vi "Video Stuff v04.vi"() -> ()   [LabVIEW 2009]
doc: "This example illustrates the use of a calibration grid to calibrate and correct an image for nonlinear distortion and accurate shape measurements.\n\nThis example loads the image of a calibration grid used to calibrate the system, learns the grid, then loads an image of parts acquired using the same setup. The example then corrects the image in two ways. The first method corrects the entire image and then measures the area of the coins. The second method corrects only the area of the coins and displays the difference in processing time."
uses:
  <vilib>/userDefined/High Color/IMAQdx.ctl
  <vilib>/vision/NI_Vision_Development_Module.lvlib
  <vilib>/vision/driver/NI_Vision_Acquisition_Software.lvlib
panel:
  out "appended array":dbl[](array[numeric])
  out "x-y":dbl[][](array[numeric])
  out "Array":i32[][](array[numeric])
  out "Small":T1(plugin-control)
  in  "Resolution":i32=36
  in  "Camera Name":T2="cam0"
  in  "Video Modes":i32(listbox)
  in  "stop":bool
  out "Live Video":T1(plugin-control)
  out "Buffer Number":u32
  in  "Red Range":cluster{"Lower value":i32, "Upper value":i32}={"Lower value"=240, "Upper value"=255}
  in  "Green Range":cluster{"Lower value":i32, "Upper value":i32}={"Lower value"=250, "Upper value"=255}
  in  "Blue Range":cluster{"Lower value":i32, "Upper value":i32}={"Lower value"=250, "Upper value"=255}
  in  "Color Mode":u16(ring) items=["RGB", "HSL", "HSV", "HSI"]
  out "Super Filter":T1(plugin-control)
  in  "Calibration File Path":path=path "C:/Documents and Settings/ekolker/My Documents/OGRE/to be synched/calibrationGrid.PNG"
  out "Top Image":T1(plugin-control) caption="Calibration Template"
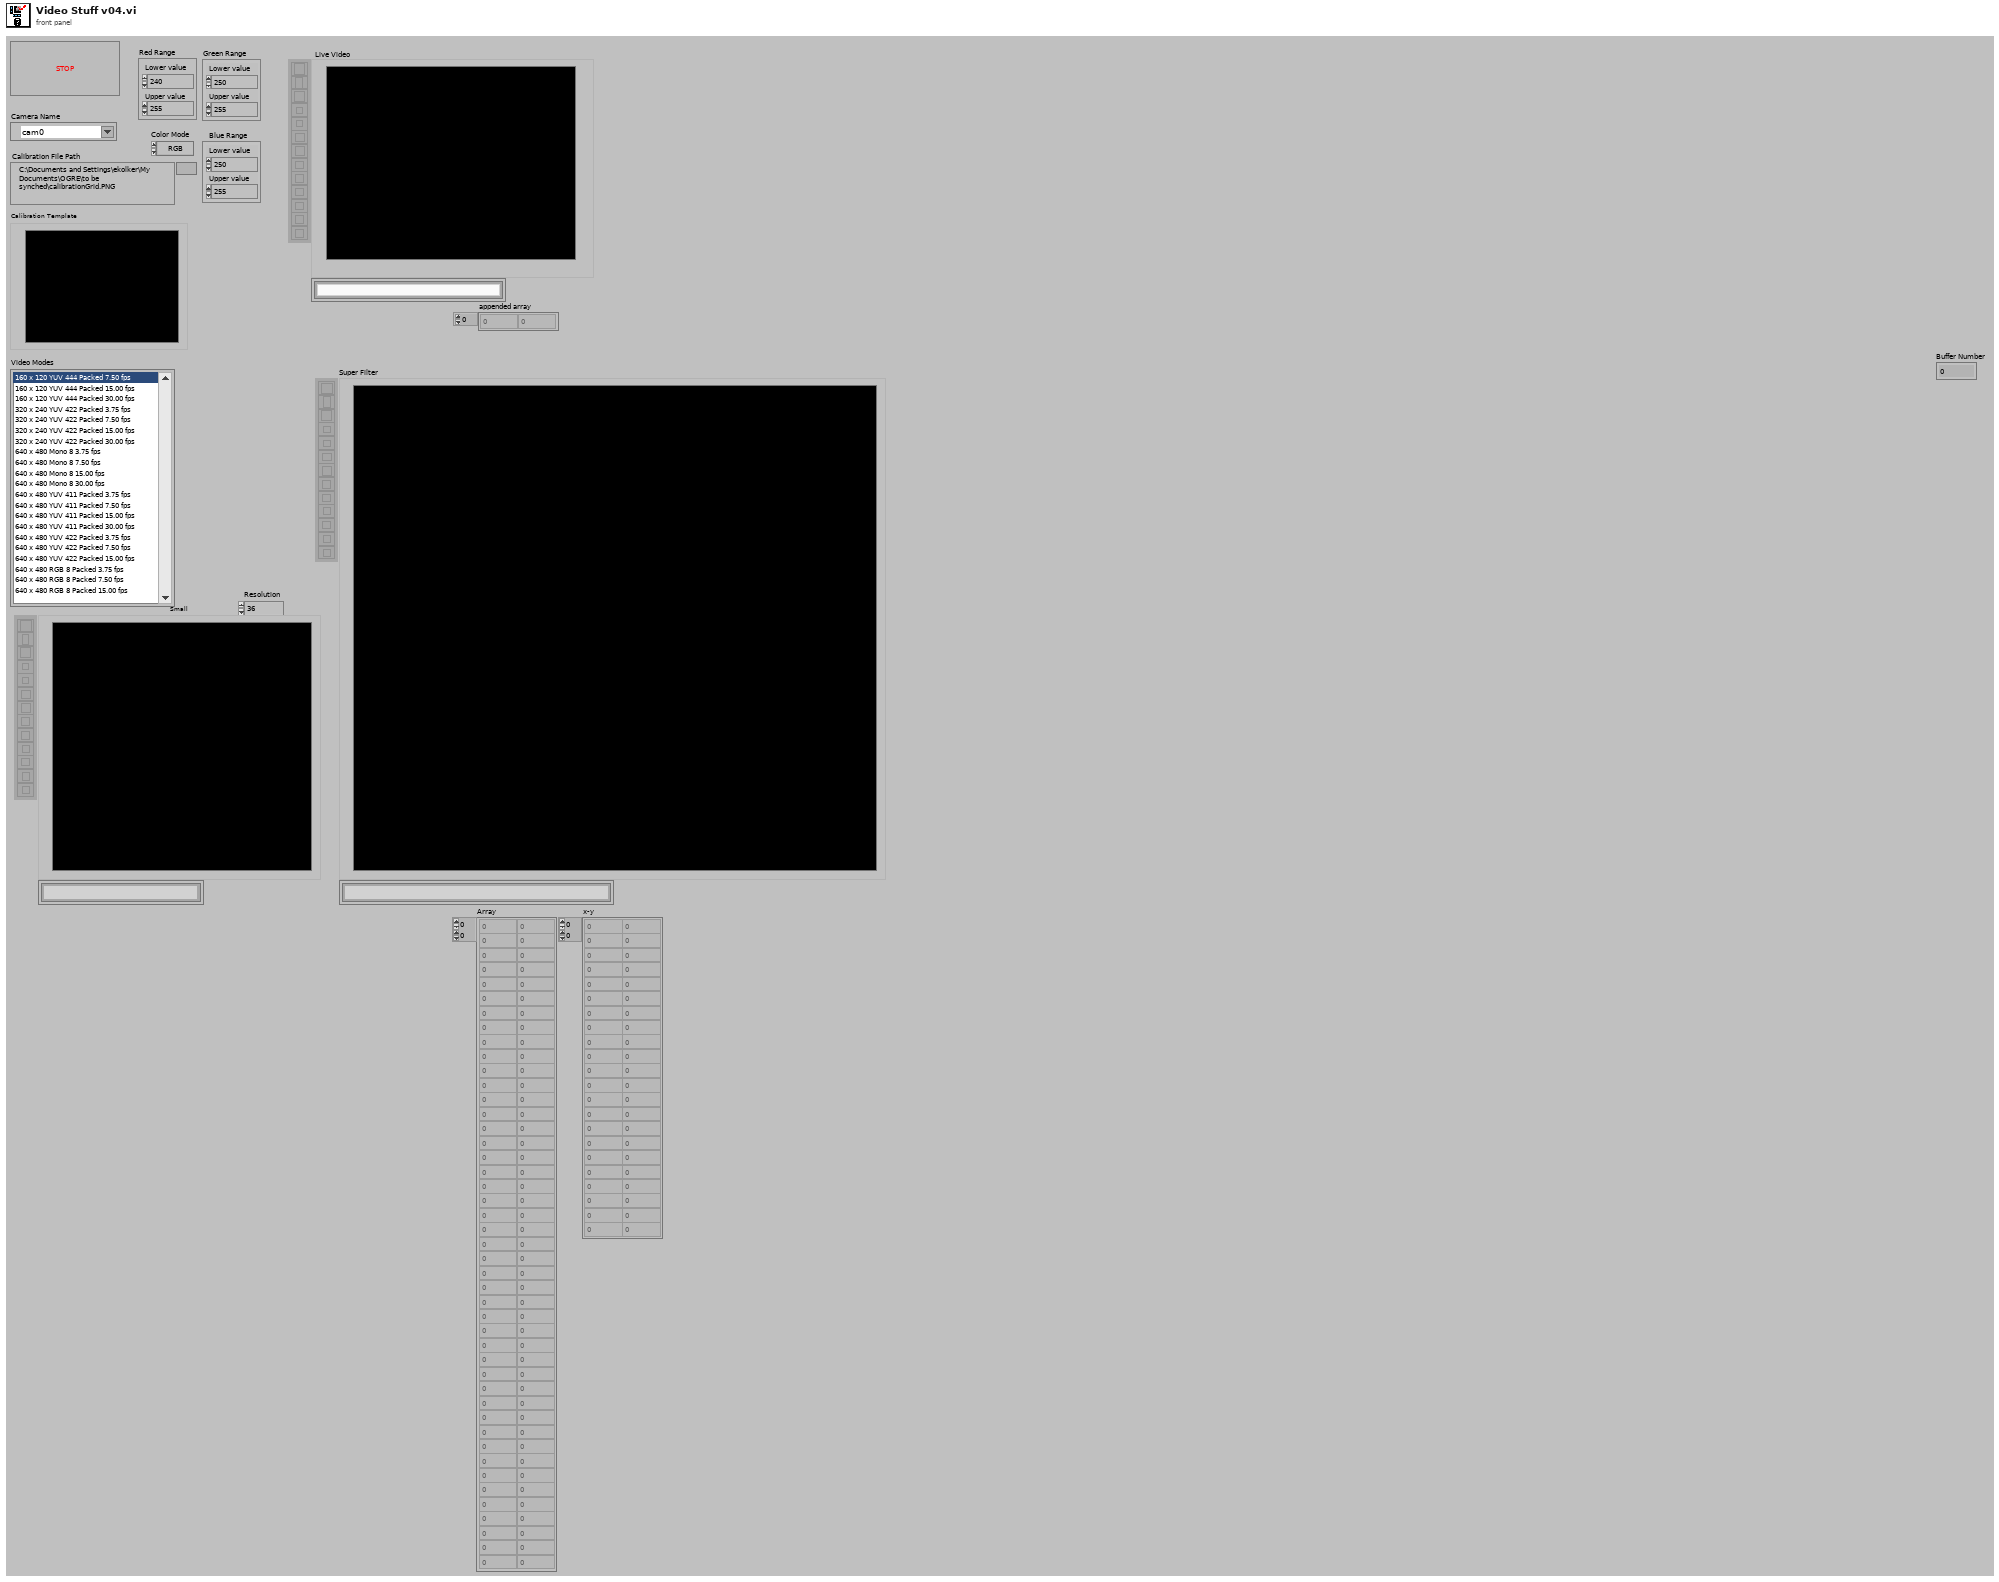
[diagram p1: front panel]
types:
  T1 = typedef "IMAQ Image.ctl" = refnum<image>
  T2 = typedef "IMAQdx.ctl" = refnum<k21>
  T3 = typedef "Image Type" = u32
  T4 = cluster{"X Step":sgl, "Y Step":sgl, "Unit":u32, "Threshold Range":cluster{"Lower value":sgl, "Upper value":sgl}}
  T5 = cluster{"Distortion":u32, "Corrected Image Scaling":u32, "Corrected Image Learn ROI":u32, "Learn Error Map?":bool, "Learn Correction Table?":bool}
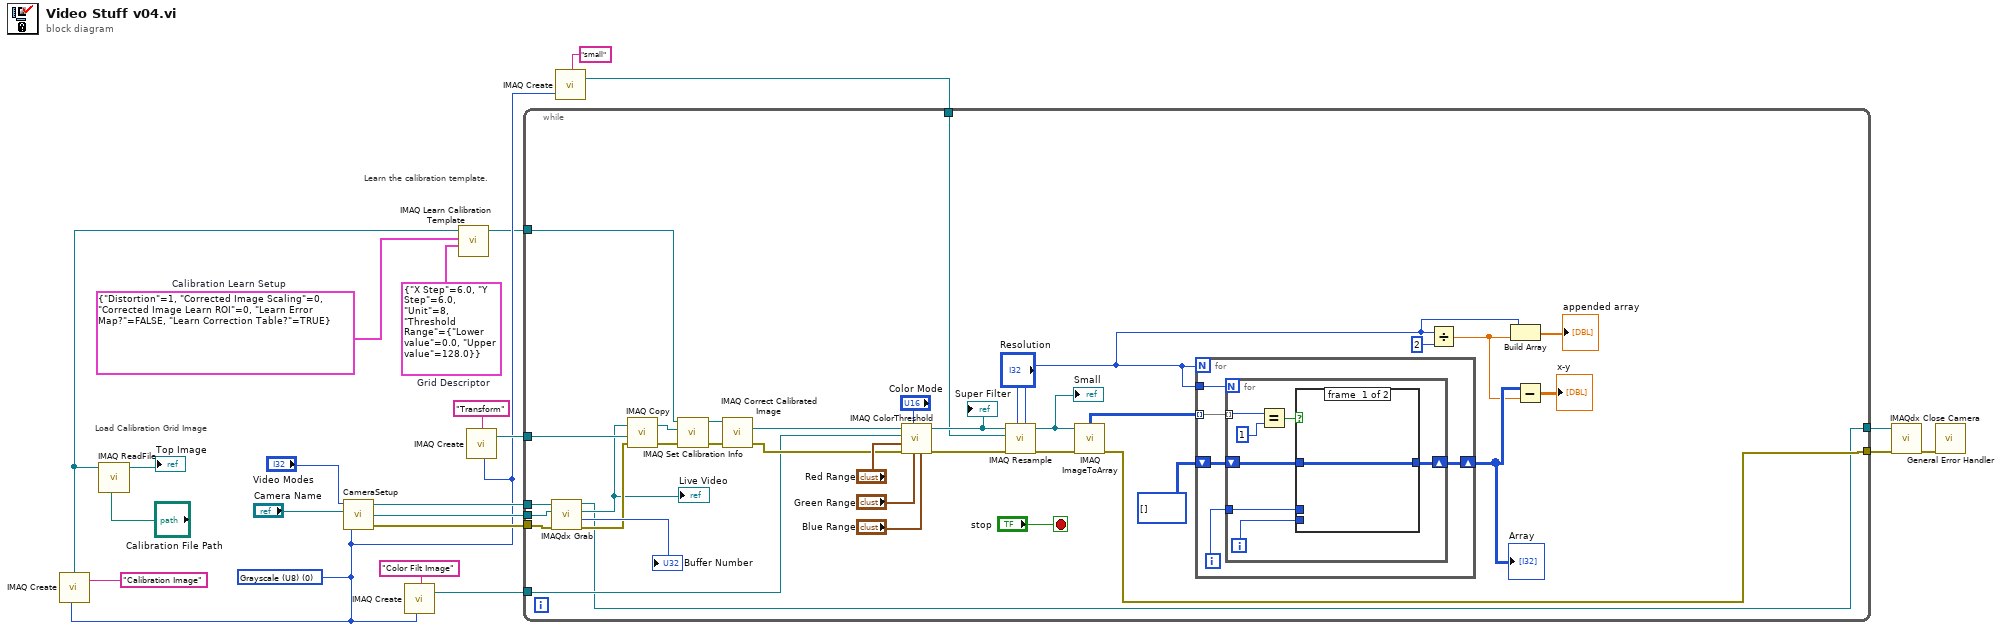
[diagram p0: block diagram]
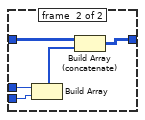
[diagram p2: hidden frame]
diagram:
  w3 = T3 0 items=["Grayscale (U8)", "Grayscale (I16)", "Grayscale (SGL)", "Complex (CSG)", "RGB (U32)", "HSL (U32)", "RGB (U64)", "Grayscale (U16)"] ("Image Type")
  w17 = T4 {"X Step"=6.0, "Y Step"=6.0, "Unit"=8, "Threshold Range"={"Lower value"=0.0, "Upper value"=128.0}}  # Grid Descriptor
  w18 = T5 {"Distortion"=1, "Corrected Image Scaling"=0, "Corrected Image Learn ROI"=0, "Learn Error Map?"=FALSE, "Learn Correction Table?"=TRUE}  # Calibration Learn Setup
  # "Load Calibration Grid Image"
  # "Learn the calibration template."
  n1 = call "IMAQ Create"("Image Name"="Calibration Image", "Image Type"=w3) -> ("New Image"=w2:T1)  [unwired: 2 in, 2 out]
  n2 = call "IMAQ ReadFile"("File Path"="Calibration File Path", "Image"=w2) -> ("Image Out"=→"Top Image":T1)  [unwired: 3 in, 6 out]
  n3 = call "CameraSetup.vi"("Image Type"=w3, "Camera Name"="Camera Name", "Video Modes"="Video Modes") -> ("error out"=w11:errorcluster, "New Image"=w6:T1, "Session Out"=w7:T2)  [unwired: 1 in]
  n4 = call "IMAQ Create"("Image Name"="Color Filt Image", "Image Type"=w3) -> ("New Image"=w20:T1)  [unwired: 2 in, 2 out]
  n5 = call "IMAQ Learn Calibration Template"("Grid Descriptor"=w17, "Calibration Learn Setup"=w18, "Image"=w2) -> ("Calibrated Image"=w1:T1)  [unwired: 4 in, 4 out]
  n6 = call "IMAQ Create"("Image Name"="Transform", "Image Type"=w3) -> ("New Image"=w19:T1)  [unwired: 2 in, 2 out]
  n7 = call "IMAQ Create"("Image Name"="small", "Image Type"=w3) -> ("New Image"=w9:T1)  [unwired: 2 in, 2 out]
  n8 = while {
    tunnel: w20 -> [w43]
    tunnel: [w30] -> w21
    tunnel: w19 -> [w49]
    tunnel: w11 -> [w44]
    tunnel: w9 -> [w31]
    tunnel: [w32] -> w8
    tunnel: w7 -> [w39]
    tunnel: w6 -> [w38]
    tunnel: w1 -> [w23]
    stop <- "stop" stop-if-true
    n9 = call <vilib>:"IMAQdx Grab.vi"("error in"=w44, "Image In"=w38, "Session In"=w39) -> ("error out"=w45:errorcluster, "Buffer Number Out"=→"Buffer Number":u32, "Image Out"=w42:T1, "Session Out"=w30:T2)  [unwired: 1 in, 4 out]
    "Live Video" <- w42
    n10 = call "IMAQ Copy"("error in (no error)"=w45, "Image Dst"=w49, "Image Src"=w42) -> ("error out"=w46:errorcluster, "Image Dst Out"=w51:T1)  [unwired: 3 in]
    n11 = call "IMAQ Set Calibration Info"("error in (no error)"=w46, "Image Dst"=w51, "Image Src"=w23) -> ("error out"=w47:errorcluster, "Calibrated Image"=w50:T1)  [unwired: 1 in, 6 out]
    n12 = call "IMAQ Correct Calibrated Image"("error in (no error)"=w47, "Image Src"=w50) -> ("error out"=w48:errorcluster, "Corrected Image"=w33:T1)  [unwired: 5 in, 3 out]
    n13 = call "IMAQ ColorThreshold"("Blue or Luma or Val or Inten Range"="Blue Range", "Green or Sat Range"="Green Range", "Color Mode"="Color Mode", "error in (no error)"=w48, "Red or Hue Range"="Red Range", "Image Dst"=w43, "Image Src"=w33) -> ("error out"=w41:errorcluster, "Image Dst Out"=w40:T1)  [unwired: 3 in]
    "Super Filter" <- w40
    n14 = call "IMAQ Resample"("X Resolution"="Resolution", "Y Resolution"="Resolution", "error in (no error)"=w41, "Image Dst"=w31, "Image Src"=w40) -> ("error out"=w37:errorcluster, "Image Dst Out"=w36:T1)  [unwired: 5 in]
    "Small" <- w36
    n15 = call "IMAQ ImageToArray"("error in (no error)"=w37, "Image"=w36) -> ("error out"=w32:errorcluster, "Image Pixels (U8)"=w35:u8[][])  [unwired: 2 in, 3 out]
    n16 = for {
      N: "Resolution" -> [_]
      tunnel: "Resolution" -> [w62]
      tunnel: w35 -> [w61] mode=indexing
      shift-right: [w60] -> w28
      shift-left: i32[][] [] -> [w59]
      i -> [w58]
      n17 = for {
        N: w62 -> [_]
        tunnel: w61 -> [w69] mode=indexing
        shift-right: [w67] -> w60
        shift-left: w59 -> [w64]
        tunnel: w58 -> [w65]
        i -> [w66]
        n18 = Equal?(x=w69, y=u8 1) -> (x = y?=w63:bool)
        n19 = case shown="True" w63 {
          tunnel: [w70 w75] -> w67
          tunnel: w66 -> [_ w74]
          tunnel: w65 -> [_ w73]
          tunnel: w64 -> [w70 w71]
          frame #0 {
          }
          frame #1 {
            n20 = Build Array(w73, w74) -> (w72:i32[])
            n21 = Build Array (concatenate)(w71, w72) -> (w75:i32[][])
          }
        }
      }
    }
    "Array" <- w28
    n22 = Divide(x="Resolution", y=2) -> (x/y=w24:dbl)
    n23 = Build Array("Resolution", w24) -> (→"appended array":dbl[])
    n24 = Subtract(x=w28, y=w24) -> (x-y=→"x-y":dbl[][])
  }
  n25 = call <vilib>:"IMAQdx Close Camera.vi"("error in"=w8, "Session In"=w21) -> ("error out"=w22:errorcluster)  [unwired: 9 out]
  n26 = call <vilib>:"General Error Handler.vi"("error in (no error)"=w22) -> ()  [unwired: 1 in, 14 out]
